vi "DAQ_Readings_from_DVS.vi"() -> ()   [LabVIEW 2013]
uses:
  <vilib>/DAQmx/read.llb/DAQmx Read (Digital Bool 1Line 1Point).vi
  <vilib>/DAQmx/read.llb/DAQmx Read (Analog 1D Wfm NChan 1Samp).vi
  <vilib>/DAQmx/miscellaneous.llb/DAQmx Fill In Error Info.vi
panel:
  out "Turbo pump on?":bool
  out "DVS DAQ Data":waveform(dbl)[](graph)
  in  "stop":bool
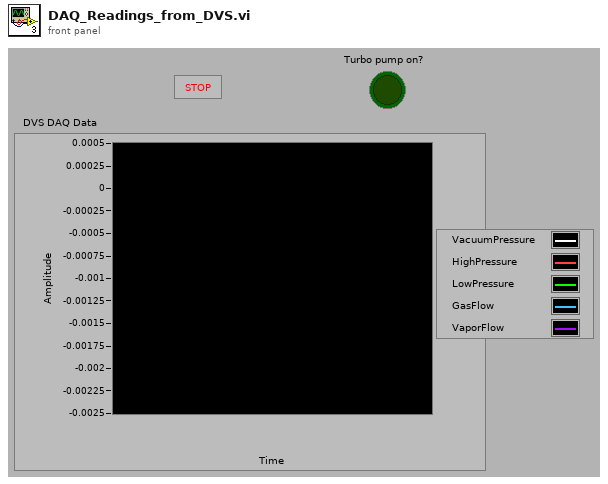
[diagram p1: front panel]
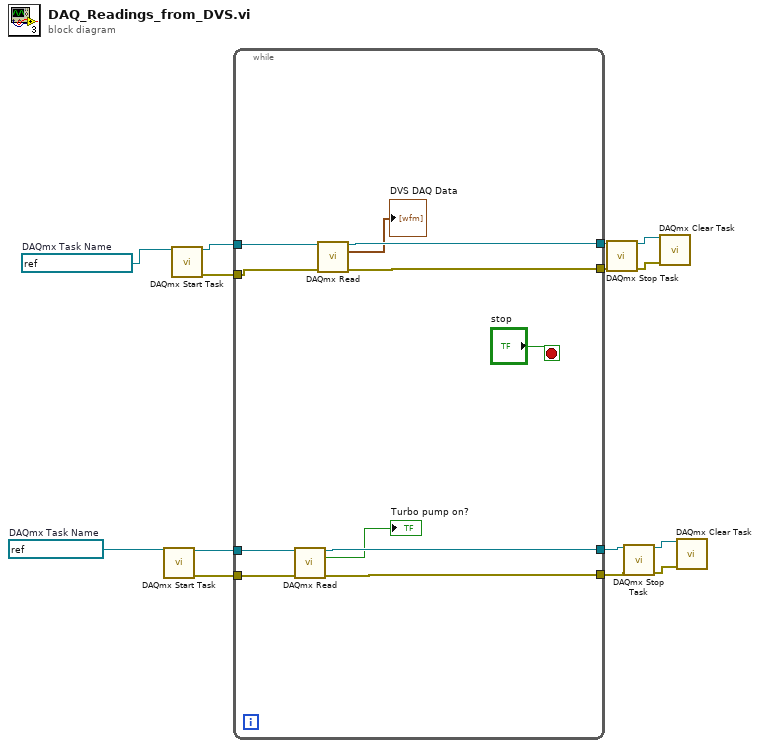
[diagram p0: block diagram]
diagram:
  w7 = refnum<k21> "Turbo Pump"  # DAQmx Task Name
  w8 = refnum<k21> "AllDaqReadings"  # DAQmx Task Name
  n1 = call <vilib>:"DAQmx Start Task.vi"("task/channels in"=w7) -> ("task out"=w2:refnum<k21>, "error out"=w1:errorcluster)  [unwired: 13 in]
  n2 = call <vilib>:"DAQmx Start Task.vi"("task/channels in"=w8) -> ("task out"=w14:refnum<k21>, "error out"=w9:errorcluster)  [unwired: 13 in]
  n3 = while {
    tunnel: w14 -> [w25]
    tunnel: [w22] -> w13
    tunnel: [w24] -> w10
    tunnel: w9 -> [w23]
    tunnel: [w20] -> w4
    tunnel: [w19] -> w3
    tunnel: w2 -> [w18]
    tunnel: w1 -> [w17]
    stop <- "stop" stop-if-true
    n4 = call-poly <vilib>:"DAQmx Read.vi"("task/channels in"=w18, "error in"=w17) -> ("task out"=w20:refnum<k21>, "data"=→"Turbo pump on?":bool, "error out"=w19:errorcluster)  [unwired: 11 in]
    n5 = call-poly <vilib>:"DAQmx Read.vi"("task/channels in"=w25, "error in"=w23) -> ("task out"=w22:refnum<k21>, "data"=→"DVS DAQ Data":waveform(dbl)[], "error out"=w24:errorcluster)  [unwired: 11 in]
  }
  n6 = call <vilib>:"DAQmx Stop Task.vi"("task/channels in"=w13, "error in"=w10) -> ("task out"=w12:refnum<k21>, "error out"=w11:errorcluster)  [unwired: 12 in]
  n7 = call <vilib>:"DAQmx Stop Task.vi"("task/channels in"=w4, "error in"=w3) -> ("task out"=w5:refnum<k21>, "error out"=w6:errorcluster)  [unwired: 12 in]
  n8 = call <vilib>:"DAQmx Clear Task.vi"("task in"=w12, "error in"=w11) -> ()  [unwired: 13 in, 1 out]
  n9 = call <vilib>:"DAQmx Clear Task.vi"("task in"=w5, "error in"=w6) -> ()  [unwired: 13 in, 1 out]
